vi "Perform Action.vi"(8 "error in":errorcluster, 10 "Input":variant, 11 "Thermometer DAQmx TC Cont CFG in":refnum<class "Thermometer DAQmx TC Cont CFG.lvclass">) -> (0 "error out":errorcluster, 2 "Output":variant, 3 "Thermometer DAQmx TC Cont CFG out":refnum<class "Thermometer DAQmx TC Cont CFG.lvclass">)   [LabVIEW 2024, in "Thermometer DAQmx TC Cont CFG.lvclass"]
uses:
  Thermometer DAQmx TC Cont CFG.lvclass
  DAQmx Base CFG/DAQmx Base CFG.lvclass/DAQmx Base CFG.ctl
  Thermometer DAQmx TC Cont CFG.lvclass/Thermometer DAQmx TC Cont CFG.ctl
  <vilib>/DAQmx/read.llb/DAQmx Read (Analog 1D Wfm NChan NSamp).vi
  <vilib>/DAQmx/miscellaneous.llb/DAQmx Fill In Error Info.vi
  DAQmx Base CFG/DAQmx Base CFG.lvclass
  Buffers/BufferLossless/BufferLossless.lvclass
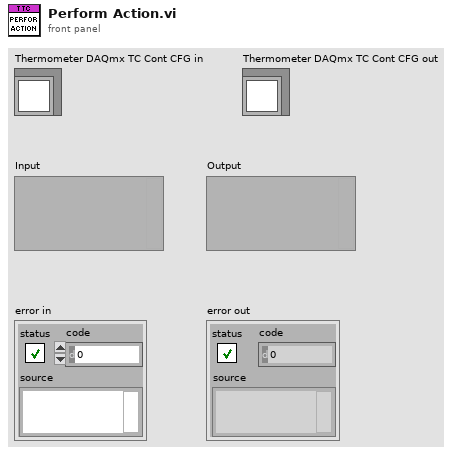
[diagram p1: front panel]
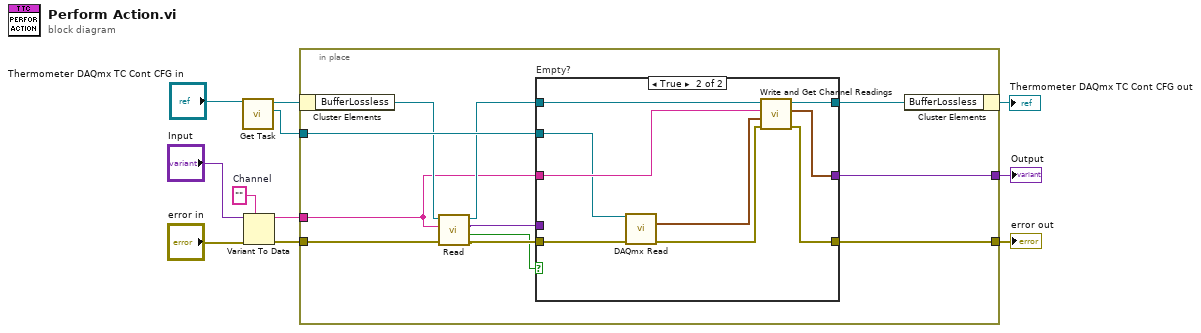
[diagram p0: block diagram]
diagram:
  w10 = ""  # Channel
  n1 = call "Get Task.vi"("DAQmx Base CFG in"="Thermometer DAQmx TC Cont CFG in") -> ("Task"=w3:refnum<k21>, "DAQmx Base CFG out"=w4:refnum<class "Thermometer DAQmx TC Cont CFG.lvclass">)  [unwired: 9 in]
  n2 = Variant To Data(error in="error in", type=w10, Variant="Input") -> (data=w6:string, error out=w7:errorcluster)
  n3 = in-place {
    in-place-border: [w22] -> w11
    in-place-border: [w21] -> w8
    in-place-border: w7 -> [w20]
    in-place-border: w6 -> [w12]
    in-place-border: w3 -> [w18]
    n4 = in-place-cluster #1(w4) -> ("BufferLossless"=w16:refnum<class "BufferLossless.lvclass">)
    n5 = call "Read.vi"("error in"=w20, "Channel"=w12, "BufferLossless in"=w16) -> ("error out"=w19:errorcluster, "empty?"=w14:bool, "Readings"=w13:variant, "BufferLossless out"=w15:refnum<class "BufferLossless.lvclass">)  [unwired: 5 in]
    n6 = case "Empty?" shown="True" w14 {
      tunnel: w19 -> [w24 w34]
      tunnel: [w24 w31] -> w22
      tunnel: [w25 w30] -> w21
      tunnel: w13 -> [w25 _]
      tunnel: w15 -> [w23 w26]
      tunnel: w12 -> [_ w33]
      tunnel: w18 -> [_ w29]
      tunnel: [w23 w28] -> w17
      frame False {
      }
      frame True {
        n7 = call-poly <vilib>:"DAQmx Read.vi"("task/channels in"=w29, "error in"=w34) -> ("data"=w27:waveform(dbl)[], "error out"=w32:errorcluster)  [unwired: 11 in, 1 out]
        n8 = call "Write and Get Channel Readings.vi"("error in"=w32, "Readings"=w27, "Channel"=w33, "BufferLossless in"=w26) -> ("error out"=w31:errorcluster, "Reading"=w30:waveform(dbl), "BufferLossless out"=w28:refnum<class "BufferLossless.lvclass">)  [unwired: 5 in]
      }
    }
    n9 = in-place-cluster #1("BufferLossless"=w17) -> (→"Thermometer DAQmx TC Cont CFG out":refnum<class "Thermometer DAQmx TC Cont CFG.lvclass">)
  }
  "error out" <- w11
  "Output" <- w8
